vi "Get Owning Ballard ARINC-429 Custom Device.vi"(8 "error in":errorcluster, 11 "item ref in":T1 format="%.0x") -> (0 "error out":errorcluster, 2 "owning Ballard ARINC-429 custom device":T1=18446744073709551615 format="%.0x", 3 "item ref out":T1 format="%.0x")   [LabVIEW 2020, in "Ballard ARINC 429 Scripting.lvlib"]
uses:
  Ballard ARINC 429 Scripting.lvlib
  <vilib>/NI VeriStand/Custom Device API/Custom Device Item Ref.ctl
  <vilib>/NI VeriStand/Custom Device Tools/Custom Device Utility Library/Search Direction.ctl
  Constants.vi
  <vilib>/NI VeriStand/Custom Device Tools/Custom Device Utility Library/NI VeriStand - Search for Item by GUID.vi
  <vilib>/NI VeriStand/Custom Device Tools/Custom Device Utility Library/Custom Device Utility Library.lvlib
  <vilib>/NI VeriStand/Custom Device API/Custom Device API.lvlib
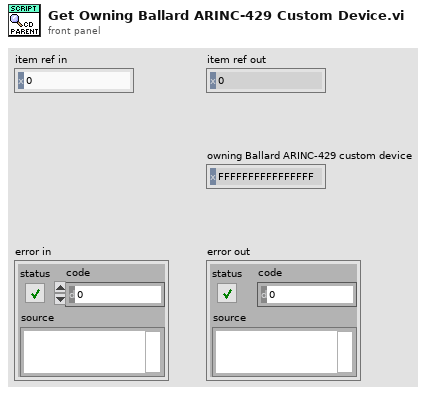
[diagram p1: front panel]
types:
  T1 = typedef "Custom Device API.lvlib/Custom Device Item Ref.ctl" = u64
  T2 = typedef "Custom Device Utility Library.lvlib/Search Direction.ctl" = enum16{"Down", "Up"}
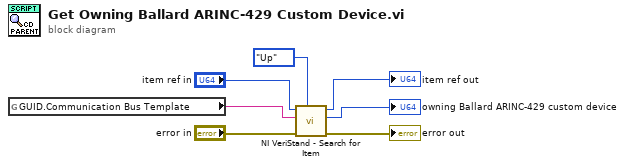
[diagram p0: block diagram]
diagram:
  n1 = global read "Constants.vi" "GUID.Communication Bus Template"() -> (w2:string)
  n2 = call-poly <vilib>:"NI VeriStand - Search for Item.vi"("Direction (Down)"=Search_Direction."Up", "error in"="error in", "Item GUID"=w2, "Section Ref in"="item ref in") -> ("error out"=→"error out":errorcluster, "Item Ref"=→"owning Ballard ARINC-429 custom device":T1, "Section Ref out"=→"item ref out":T1)  [unwired: 4 in, 1 out]
